vi "Actor Core.vi"(8 "error in":errorcluster, 11 "Elevator Controller in":refnum<class "Sim Sensor Interface Actor.lvclass">) -> (0 "error out":errorcluster, 3 "Actor out":refnum<class "Actor.lvclass">)   [LabVIEW 2019, in "Sim Sensor Interface Actor.lvlib" / "Sim Sensor Interface Actor.lvclass"]
doc: "(<B>Filename</B>: Actor Framework.lvlib:Actor.lvclass:Actor Core.vi)\n\nReceives messages to the actor, reacts to them, and initiates any error handling that may shut the actor down.\n\nDescendant classes may override this VI to append parallel tasks for the actor to complete while it handles messages. Overrides use the Call Parent Method node."
uses:
  Sim Sensor Interface Actor.lvclass
  <vilib>/ActorFramework/Actor/Actor.lvclass
  <vilib>/ActorFramework/Stop Msg/Stop Msg.lvclass
  Sensor Interface Actor/Sensor Interface Actor/Sensor Interface Actor.lvclass
  Elevator Controller/Elevator Controller Messages/Set Enable Door Buttons Msg/Set Enable Door Buttons Msg.lvclass
  C:/Workspace/CLA/Elevator AF 3rd/Sensor Interface Actor/Sensor Interface Actor/Sensor Interface Actor.lvclass
  C:/Program Files (x86)/National Instruments/LabVIEW 2019/vi.lib/ActorFramework/Actor/Actor.lvclass
panel:
  out "Elevator Position":u8(slide) scale=1.0..4.0
  # "[Covers: UI4]"
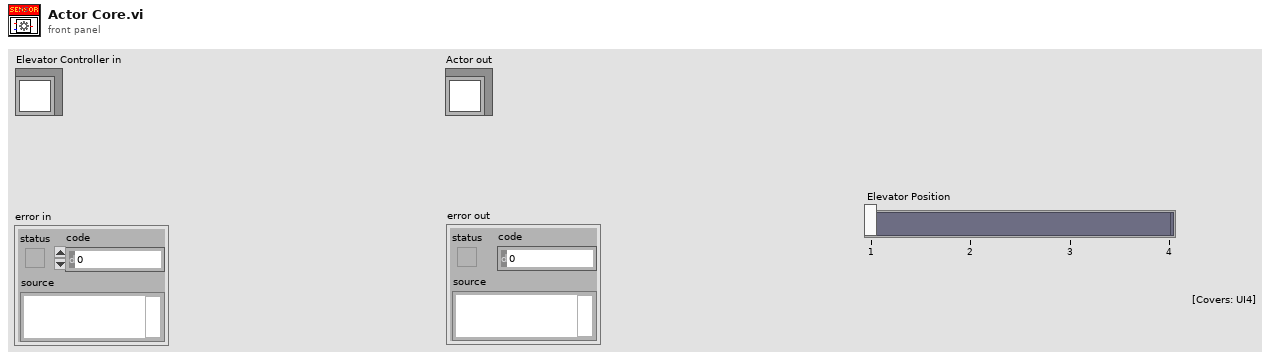
[diagram p1: front panel]
types:
  T1 = enum8{"Enabled", "Disabled", "Disabled and Grayed Out"}
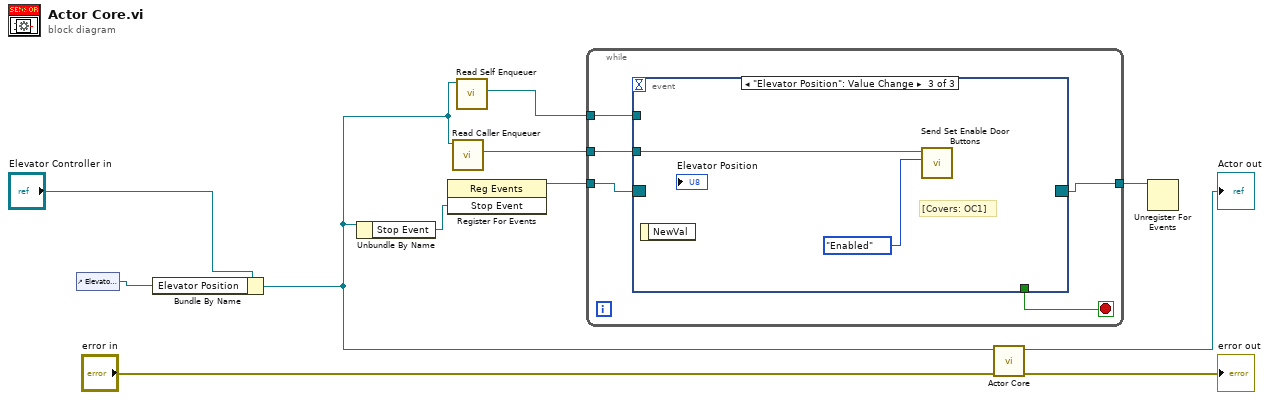
[diagram p0: block diagram]
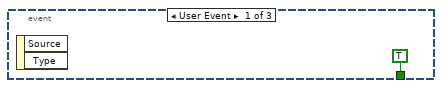
[diagram p2: hidden frame]
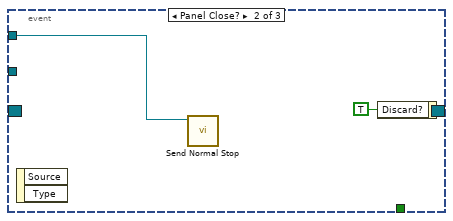
[diagram p3: hidden frame]
diagram:
  n1 = control-ref of="Elevator Position"() -> (w3:refnum<vi>)
  n2 = Bundle By Name(cluster="Elevator Controller in", "Elevator Position"=w3) -> (w2:refnum<class "Sim Sensor Interface Actor.lvclass">)
  n3 = Unbundle By Name(w2) -> ("Stop Event"=w6:refnum<user-event>)
  n4 = register-events(w6) -> (reference out=w8:refnum<event-registration>)  [unwired: 2 in, 1 out]
  n5 = call <vilib>:"Read Caller Enqueuer.vi"("Actor"=w2) -> ("Caller Enqueuer"=w1:refnum<class "Message Enqueuer.lvclass">)  [unwired: 10 in]
  n6 = call <vilib>:"Read Self Enqueuer.vi"("Actor"=w2) -> ("Self Enqueuer"=w5:refnum<class "Message Enqueuer.lvclass">)  [unwired: 10 in]
  n7 = while {
    tunnel: w8 -> [w16]
    tunnel: [w15] -> w7
    tunnel: w5 -> [w14]
    tunnel: w1 -> [w12]
    stop <- w13 stop-if-true
    n8 = event shown="[2] \"Elevator Position\": Value Change" {
      selector: w16 -> [_ _ _]
      dyn-events: [_ _ _] -> w15
      timeout: _ -> [_ _ _]
      tunnel: w14 -> [_ w18 _]
      tunnel: [TRUE _ _] -> w13
      tunnel: w12 -> [_ _ w21]
      event User Event {
        n9 = event-data() -> ()  [unwired: 1 in, 2 out]
      }
      event Panel Close? {
        n10 = event-data() -> ()  [unwired: 1 in, 2 out]
        n11 = call <vilib>:"Send Normal Stop.vi"("Message Enqueuer"=w18) -> ()  [unwired: 10 in, 1 out]
        n12 = event-data("Discard?"=TRUE) -> ()  [unwired: 1 in, 1 out]
      }
      event "Elevator Position": Value Change {
        # "[Covers: OC1]"
        n13 = event-data() -> ()  [unwired: 1 in, 1 out]
        n14 = call "Send Set Enable Door Buttons.vi"("Disabled"=T1."Enabled", "Message Enqueuer"=w21) -> ()  [unwired: 8 in, 2 out]
      }
    }
  }
  n15 = call-parent "Actor Core.vi"("error in"="error in", "Actor in"=w2) -> ("error out"=→"error out":errorcluster, "Actor out"=→"Actor out":refnum<class "Actor.lvclass">)  [unwired: 8 in]
  n16 = Unregister For Events(event registration refnum=w7) -> ()  [unwired: 1 in, 1 out]
